vi "Get Image.vi"(8 "error in (no error)":errorcluster, 10 "Image Name":string, 11 "Item Ref out out":T2 format="%.0x") -> (0 "error out":errorcluster, 1 "Loaded Image Data (float)":sgl[][](array[numeric]), 2 "Image out":T1, 3 "Item Ref out":T2 format="%.0x")   [LabVIEW 2011, in "Meter Detection Custom Device.lvlib"]
uses:
  Meter Detection Custom Device.lvlib
  <vilib>/NI Veristand/Custom Device API/Custom Device Item Ref.ctl
  <vilib>/vision/Image Controls.llb/IMAQ Image.ctl
  Meter Detection Global Variable.vi
  <vilib>/NI Veristand/Custom Device API/Get Item Property (Variant).vi
  <vilib>/NI Veristand/Custom Device API/Custom Device API.lvlib
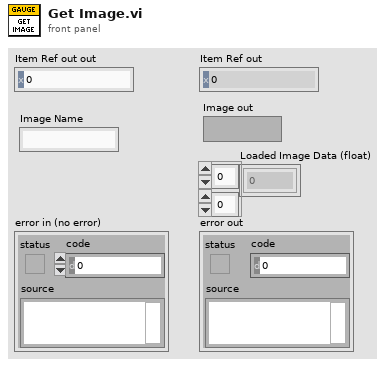
[diagram p1: front panel]
types:
  T1 = typedef "IMAQ Image.ctl" = refnum<image>
  T2 = typedef "Custom Device API.lvlib/Custom Device Item Ref.ctl" = u64
  T3 = typedef "Image Type" = u32
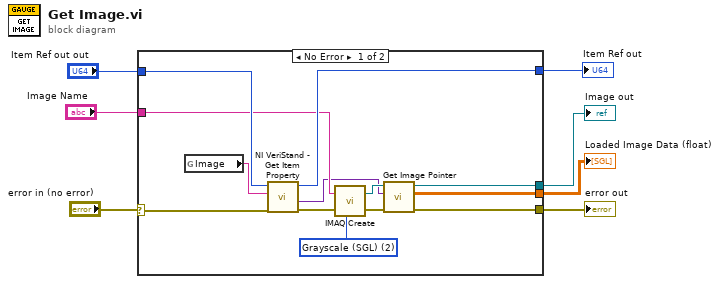
[diagram p0: block diagram]
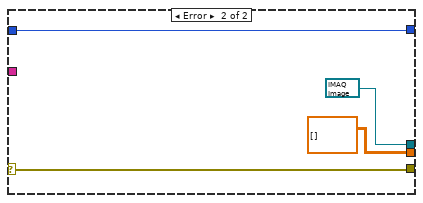
[diagram p2: hidden frame]
diagram:
  n1 = case shown="No Error" "error in (no error)" {
    selector: "error in (no error)" -> [w8 w23]
    tunnel: [w20 w24] -> w7
    tunnel: "Item Ref out out" -> [w18 w24]
    tunnel: "Image Name" -> [w14 _]
    tunnel: [w11 w23] -> w4
    tunnel: [w10 T1 refnum ("Image out")] -> w3
    tunnel: [w9 sgl[][] [] ("Loaded Image Data (float)")] -> w2
    frame No Error {
      w15 = T3 2 items=["Grayscale (U8)", "Grayscale (I16)", "Grayscale (SGL)", "Complex (CSG)", "RGB (U32)", "HSL (U32)", "RGB (U64)", "Grayscale (U16)"] ("Image Type")
      n2 = global read "Meter Detection Global Variable.vi" "Image"() -> (w19:string)
      n3 = call-poly <vilib>:"NI VeriStand - Get Item Property.vi"("error in (no error)"=w8, "Property Name"=w19, "Item Ref in"=w18) -> ("error out"=w12:errorcluster, "Value"=w13:variant, "Item Ref out"=w20:T2)  [unwired: 5 in, 1 out]
      n4 = call "IMAQ Create"("Image Name"=w14, "Image Type"=w15, "error in (no error)"=w12) -> ("New Image"=w16:T1, "error out"=w17:errorcluster)  [unwired: 2 in]
      n5 = call "Get Image Pointer.vi"("error in (no error)"=w17, "Image Data"=w13, "Image in"=w16) -> ("error out"=w11:errorcluster, "Loaded Image Data (float)"=w9:sgl[][], "Image out"=w10:T1)  [unwired: 6 in]
    }
    frame Error {
    }
  }
  "Item Ref out" <- w7
  "error out" <- w4
  "Image out" <- w3
  "Loaded Image Data (float)" <- w2
